vi "Build all.vi"() -> ()   [LabVIEW 2021]
uses:
  <vilib>/JKI/VIPM API/command-line/support/VI Package Build Spec Data Cluster_vipm_api.ctl
  <vilib>/JKI/VIPM API/command-line/support/Version Info Cluster_vipm_api.ctl
  <vilib>/JKI/VIPM API/VIPM API_vipm_api.lvlib
panel:
  out "VI Package Build Spec Data":T1
  out "appended array":string[](array[string])
  out "Build time":dbl
  out "error out":errorcluster
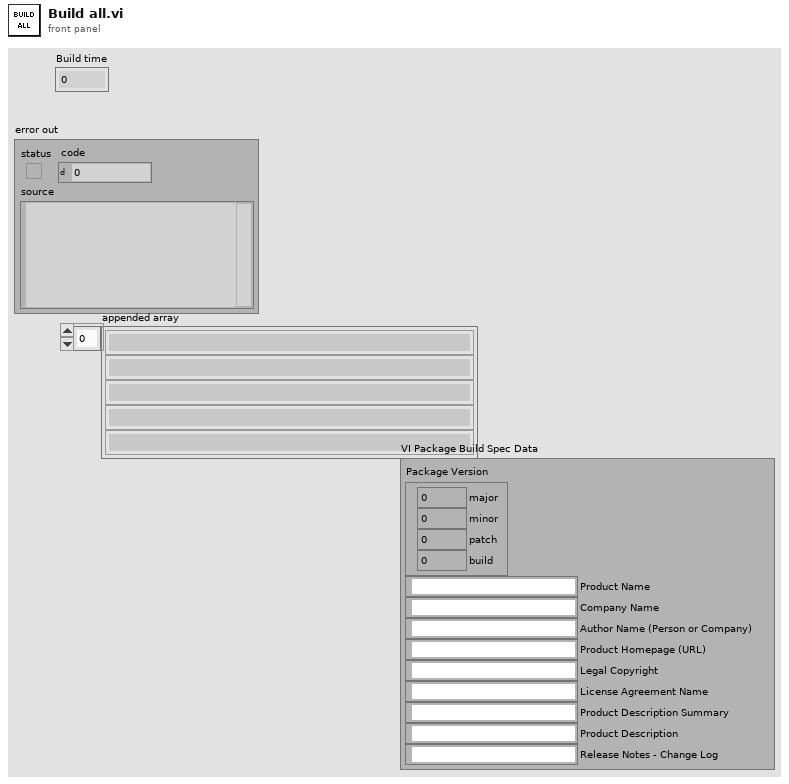
[diagram p1: front panel]
types:
  T1 = typedef "VIPM API_vipm_api.lvlib/VI Package Build Spec Data Cluster_vipm_api.ctl" = cluster{"Package Version":T2, "Product Name":string, "Company Name":string, "Author Name (Person or Company)":string, "Product Homepage (URL)":string, "Legal Copyright":string, "License Agreement Name":string, "Product Description Summary":string, "Product Description":string, "Release Notes - Change Log":string}
  T2 = typedef "VIPM API_vipm_api.lvlib/Version Info Cluster_vipm_api.ctl" = cluster{"major":u32, "minor":u32, "patch":u32, "build":u32}
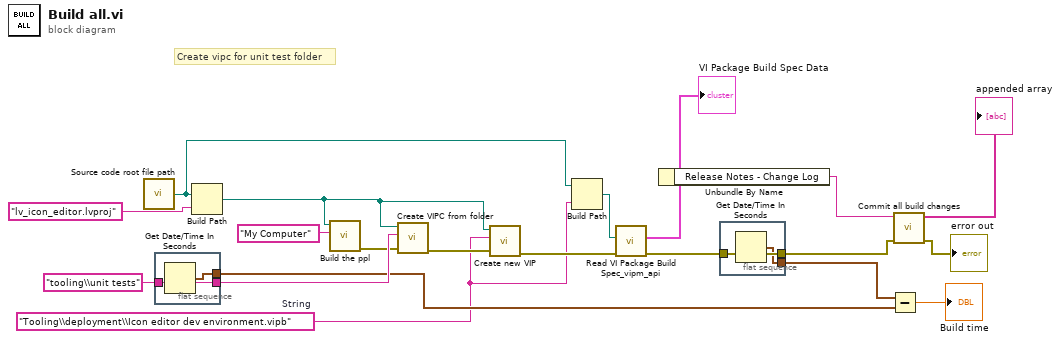
[diagram p0: block diagram]
diagram:
  w5 = "Tooling\\deployment\\Icon editor dev environment.vipb"  # String
  # "Create vipc for unit test folder"
  n1 = call "Source code root file path.vi"() -> ("Source code root path"=w6:path)  [unwired: 1 in]
  n2 = flat-sequence {
    tunnel: "tooling\\unit tests" ("Dependency folder relative path") -> [w22]
    tunnel: [w22] -> w18
    tunnel: [w21] -> w16
    frame #0 {
      n3 = Get Date/Time In Seconds() -> (seconds since 1Jan1904=w21:timestamp)
    }
  }
  n4 = Build Path(base path=w6, name or relative path="lv_icon_editor.lvproj" ("Dependency folder relative path")) -> (appended path=w9:path)
  n5 = call "Build the ppl.vi"("Name of target (My Computer)"="My Computer", "Path override"=w9) -> ("error out"=w10:errorcluster)  [unwired: 8 in, 1 out]
  n6 = call "Create VIPC from folder.vi"("error in (no error)"=w10, "Dependency folder relative path"=w18, "Project path"=w9) -> ("error out"=w11:errorcluster)  [unwired: 8 in]
  n7 = call "Create new VIP.vi"("error in (no error)"=w11, "String"=w5, "Project path"=w9) -> ("error out"=w8:errorcluster)  [unwired: 7 in, 1 out]
  n8 = Build Path(base path=w6, name or relative path=w5) -> (appended path=w4:path)
  n9 = call <vilib>:"Read VI Package Build Spec_vipm_api.vi"("error in (no error)"=w8, "Path to VIPB File"=w4) -> ("error out"=w7:errorcluster, "VI Package Build Spec Data"=w3:T1)  [unwired: 8 in]
  "VI Package Build Spec Data" <- w3
  n10 = Unbundle By Name(w3) -> ("Release Notes - Change Log"=w2:string)
  n11 = flat-sequence {
    tunnel: w7 -> [w24]
    tunnel: [w24] -> w14
    tunnel: [w23] -> w17
    frame #0 {
      n12 = Get Date/Time In Seconds() -> (seconds since 1Jan1904=w23:timestamp)
    }
  }
  n13 = Subtract(x=w17, y=w16) -> (x-y=→"Build time":dbl)
  n14 = call "Commit all build changes.vi"("error in"=w14, "msg"=w2) -> ("error out"=→"error out":errorcluster, "appended array"=→"appended array":string[])  [unwired: 8 in]
